vi "Evaluate.vi"(0 "object in":refnum<class "nsei.lvclass">, 1 "Game":refnum<class "Game.lvclass">, 2 "Point":dbl[](array[numeric]), 3 "Ally?":bool, 5 "error in (no error)":errorcluster) -> (14 "object out":refnum<class "nsei.lvclass">, 16 "Evaluation":dbl, 19 "error out":errorcluster)   [LabVIEW 2023, in "nsei.lvclass"]
uses:
  nsei.lvclass
  Criterion_class/Criterion.lvclass
  Game_class/Game.lvclass
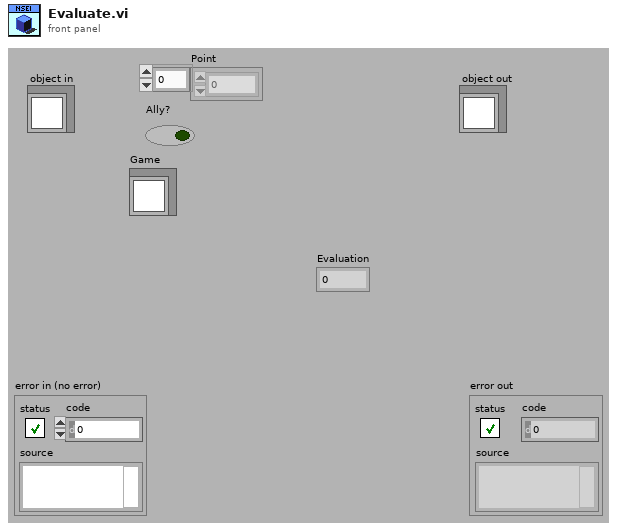
[diagram p1: front panel]
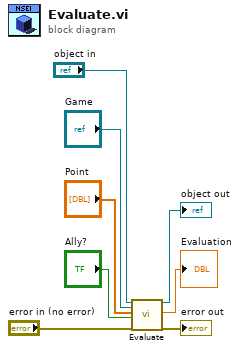
[diagram p0: block diagram]
diagram:
  n1 = call-parent "Evaluate.vi"("object in"="object in", "Game"="Game", "Point"="Point", "Ally?"="Ally?", "error in (no error)"="error in (no error)") -> ("object out"=→"object out":refnum<class "nsei.lvclass">, "Evaluation"=→"Evaluation":dbl, "error out"=→"error out":errorcluster)  [unwired: 12 in]
